vi "Infinite Message Manager - Core.vi"(6 "Infinite Message Selector":T1, 7 "Msg ID":string, 8 "error in (no error)":errorcluster, 9 "Tau parameter":string, 10 "Actor Framework:Message":refnum<class "Message.lvclass">, 11 "Ancestor in":refnum<class "Ancestor.lvclass">) -> (0 "error out":errorcluster, 2 "Exists?":bool, 3 "Ancestor out":refnum<class "Ancestor.lvclass">)   [LabVIEW 2026, in "TALOS.lvlib" / "Ancestor.lvlib" / "Ancestor.lvclass"]
doc: "This VI start the infinite messaging to periodically check the message given in input. It grabs the notifier so to be able to stop it afterwards."
uses:
  Ancestor.lvclass
  builds/Actor Framework PPL/Actor Framework.lvlibp/1abvi3w/vi.lib/ActorFramework/Message/Message.lvclass
  C:/LabVIEW Code/TALOS/builds/Actor Framework PPL/Actor Framework.lvlibp/1abvi3w/vi.lib/ActorFramework/Actor/Actor.lvclass
  Infinite Message Selector.ctl
  Ancestor.lvclass/Ancestor.ctl
  builds/Actor Framework PPL/Actor Framework.lvlibp/1abvi3w/vi.lib/ActorFramework/Time-Delayed Send Message/Time-Delay Override Options.ctl
  FGV/Error Memory/Get Error Description.vi
  Support VIs/Get PC name.vi
  Read ID.vi
  Support VIs/Get Class Name.vi
  Support VIs/Circus Root Path.vi
  FGV/Error Memory/Error Memory Core.vi
  <vilib>/AdvancedString/Delimited String to 1D String Array.vi
  <vilib>/AdvancedString/Delimited String to 1D String Array (string).vi
  FGV/Error Memory/Error Crt Lvl checker.vi
  FGV/Error Memory/Error Memory Core.vi/40c8088d-b597-4017-91af-faa98e00292e.vi
  FGV/Error Memory/Error Memory Core.vi/d4a3ab98-063c-4e44-b43d-fbdcfe6c2be2.vi
  Support VIs/Global Memory.vi
  <vilib>/Utility/LVClass/Get LV Class Name.vi
  Support VIs/Is in Packed Library.vi
  Support VIs/TALOS Root path.vi
  Support VIs/Read CSV worksheet.vi
  Support VIs/Global Constants.vi
  <vilib>/Utility/error.llb/General Error Handler.vi
  <vilib>/Utility/config.llb/Open Config Data.vi
  <vilib>/Utility/config.llb/Get Section Names.vi
  <vilib>/Utility/config.llb/Get Key Names.vi
  <vilib>/Utility/config.llb/Read Key.vi
  <vilib>/Utility/config.llb/Read Key (String).vi
  <vilib>/Utility/config.llb/Close Config Data.vi
  Support VIs/Error Log.vi
  <vilib>/Comparison/Equal/Equal Functor/Equal Functor.lvclass
  builds/Actor Framework PPL/Actor Framework.lvlibp
  builds/Actor Framework PPL/Actor Framework.lvlibp/1abvi3w/vi.lib/ActorFramework/Actor/Actor.lvclass
  TALOS.lvlib
  <userlib>/_OpenG.lib/lvdata/lvdata.llb/openg_variant.lvlib
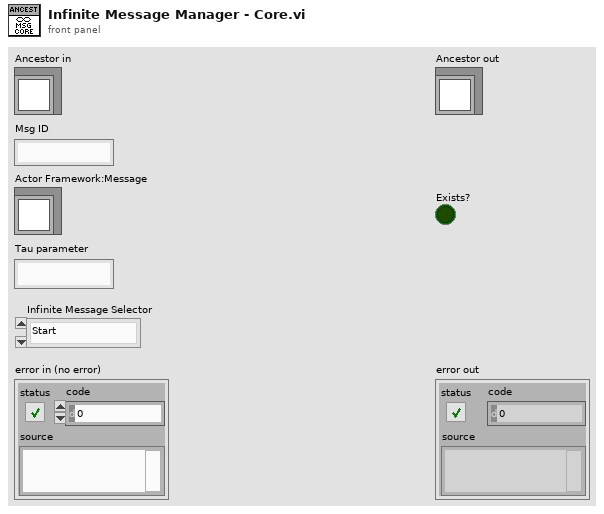
[diagram p1: front panel]
types:
  T1 = typedef "TALOS.lvlib/Ancestor.lvlib/Ancestor.lvclass/Infinite Message Selector.ctl" = enum16{"Start", "Stop", "Check", "Flush (Stop all)", "Init"}
  T2 = typedef "Actor Framework.lvlibp/Time-Delay Override Options.ctl" = enum16{"Send next copy now", "Skip next scheduled copy", "Send next copy now and stop all further copies", "Stop all further copies"}
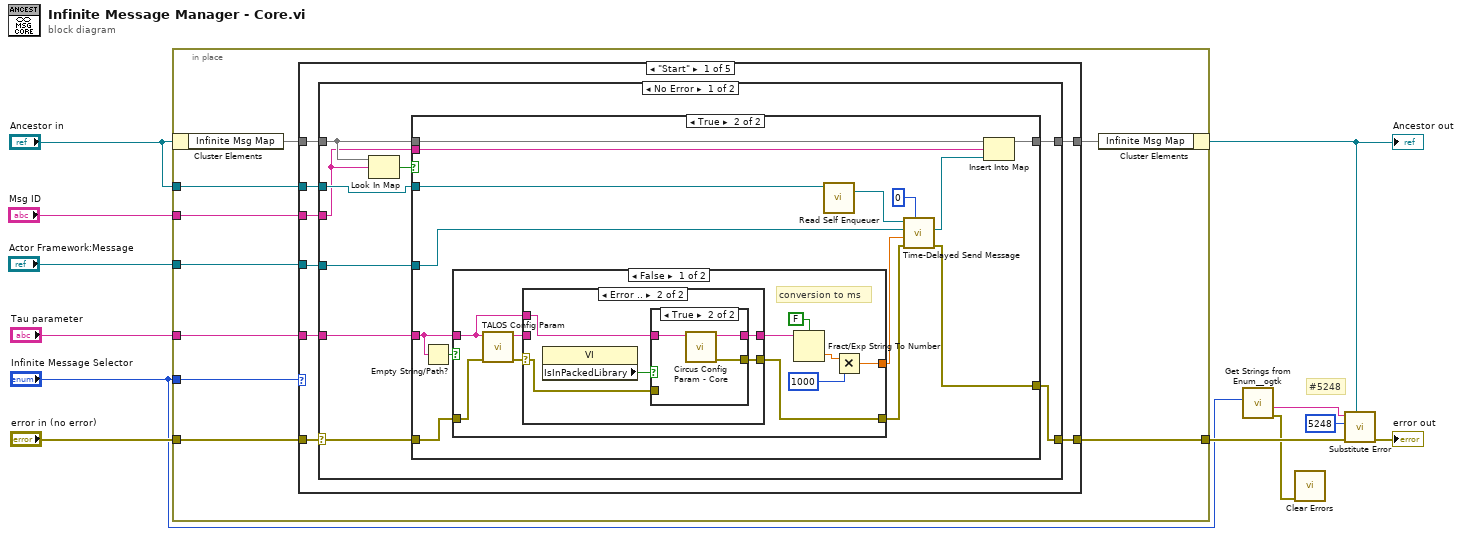
[diagram p0: block diagram]
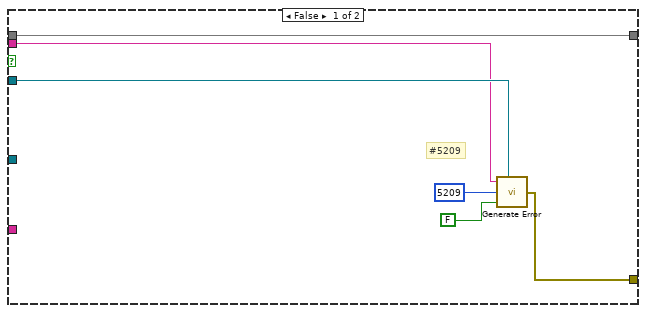
[diagram p2: hidden frame]
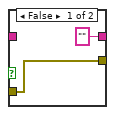
[diagram p4: hidden frame]
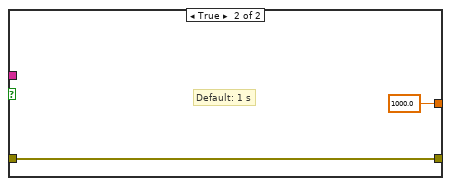
[diagram p5: hidden frame]
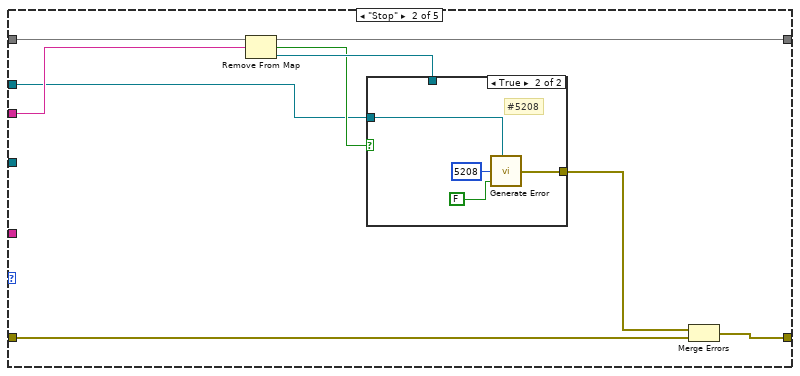
[diagram p7: hidden frame]
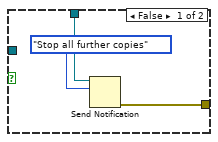
[diagram p8: hidden frame]
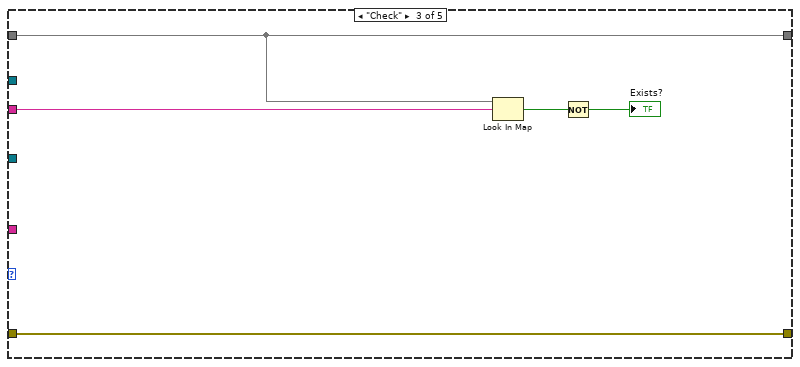
[diagram p9: hidden frame]
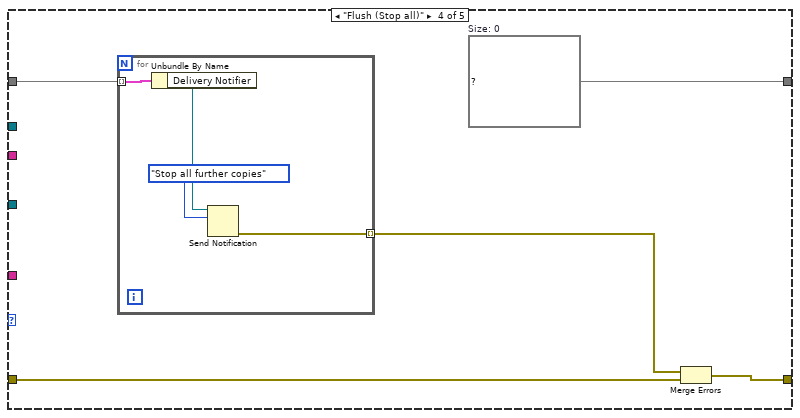
[diagram p10: hidden frame]
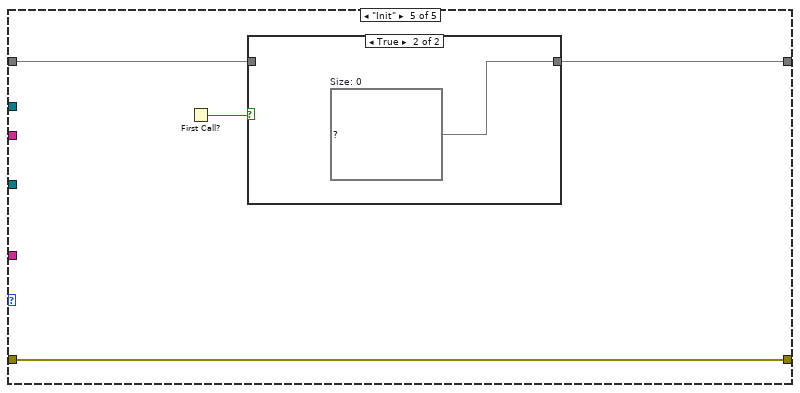
[diagram p11: hidden frame]
diagram:
  # "#5248"
  n1 = in-place {
    in-place-border: "error in (no error)" -> [w13]
    in-place-border: "Actor Framework:Message" -> [w14]
    in-place-border: "Tau parameter" -> [w21]
    in-place-border: "Infinite Message Selector" -> [w20]
    in-place-border: [w19] -> w7
    in-place-border: "Ancestor in" -> [w16]
    in-place-border: "Msg ID" -> [w15]
    n2 = in-place-cluster #1("Ancestor in") -> ("Infinite Msg Map"=w18:map{string, refnum<notifier>})
    n3 = case shown="\"Start\"" w20 {
      tunnel: w16 -> [w29 w87 _ _ _]
      tunnel: [w28 w86 w101 w107 w117] -> w19
      tunnel: [w25 w92 w105 w109 w118] -> w17
      tunnel: w18 -> [w23 w91 w105 w110 w115]
      tunnel: w14 -> [w26 _ _ _ _]
      tunnel: w21 -> [w27 _ _ _ _]
      tunnel: w15 -> [w22 w88 w104 _ _]
      tunnel: w13 -> [w24 w85 w101 w106 w117]
      frame "Start" {
        n4 = case shown="No Error" w24 {
          selector: w24 -> [w33 w84]
          tunnel: w29 -> [w38 _]
          tunnel: [w37 w84] -> w28
          tunnel: w27 -> [w36 _]
          tunnel: w26 -> [w35 _]
          tunnel: [w34 w83] -> w25
          tunnel: w23 -> [w32 w83]
          tunnel: w22 -> [w31 _]
          frame No Error {
            n5 = Look In Map(map=w32, key=w31) -> (key not found?=w30:bool)  [unwired: 1 in, 1 out]
            n6 = case shown="True" w30 {
              tunnel: w38 -> [w40 w55]
              tunnel: [w41 w54] -> w37
              tunnel: w36 -> [_ w45]
              tunnel: w35 -> [_ w53]
              tunnel: [w44 w51] -> w34
              tunnel: w33 -> [_ w50]
              tunnel: w32 -> [w44 w49]
              tunnel: w31 -> [w39 w48]
              frame False {
                # "#5209"
                n7 = call "Generate Error.vi"("Optional String"=w39, "Class"=w40, "Error Code"=5209, "Error/Warning"=FALSE) -> ("error out"=w41:errorcluster)  [unwired: 3 in]
              }
              frame True {
                n8 = Empty String/Path?(string/path=w45) -> (empty?=w46:bool)
                n9 = case shown="False" w46 {
                  tunnel: [w68 1000.0] -> w57
                  tunnel: w50 -> [w66 w82]
                  tunnel: [w63 w82] -> w47
                  tunnel: w45 -> [w62 _]
                  frame False {
                    # "conversion to ms"
                    n10 = call "TALOS Config Param.vi"("error in (no error)"=w66, "Parameter Name"=w62) -> ("error out"=w65:errorcluster, "Output"=w64:string)  [unwired: 8 in]
                    n11 = case shown="Error .." w65 {
                      selector: w65 -> [w70 w73]
                      tunnel: w64 -> [w69 _]
                      tunnel: [w70 w72] -> w63
                      tunnel: [w69 w74] -> w61
                      tunnel: w62 -> [_ w71]
                      frame No Error {
                      }
                      frame Error {
                        n12 = property class="VI"() -> ("IsInPackedLibrary"=w75:bool)  [unwired: 2 in, 2 out]
                        n13 = case shown="True" w75 {
                          tunnel: ["" ("Output") w79] -> w74
                          tunnel: w73 -> [w77 _]
                          tunnel: [w77 w80] -> w72
                          tunnel: w71 -> [_ w78]
                          frame False {
                          }
                          frame True {
                            n14 = call "Circus Config Param - Core.vi"("Parameter Name"=w78) -> ("error out"=w80:errorcluster, "Output"=w79:string)  [unwired: 9 in]
                          }
                        }
                      }
                    }
                    n15 = Fract/Exp String To Number(use system decimal point (T)=FALSE, string=w61) -> (number=w60:dbl)  [unwired: 2 in, 1 out]
                    n16 = Multiply(x=w60, y=1000) -> (x*y=w68:dbl)
                  }
                  frame True {
                    # "Default: 1 s"
                  }
                }
                n17 = call "Read Self Enqueuer.vi"("Actor"=w55) -> ("Self Enqueuer"=w56:refnum<class "Message Enqueuer.lvclass">)  [unwired: 10 in]
                n18 = call "Time-Delayed Send Message.vi"("# Copies (0 = infinite repeat)"=u32 0, "error in (no error)"=w47, "Milliseconds To Wait"=w57, "Message"=w53, "Message Enqueuer"=w56) -> ("error out"=w54:errorcluster, "Delivery Notifier"=w52:refnum<notifier>)  [unwired: 5 in]
                n19 = Insert Into Map(map in=w49, key=w48, value=w52) -> (map out=w51:map{string, refnum<notifier>})  [unwired: 2 out]
              }
            }
          }
          frame Error {
          }
        }
      }
      frame "Stop" {
        n20 = Remove From Map(10:w88, 11:w91) -> (1:w90:refnum<notifier>, 2:w89:bool, 3:w92:map{string, refnum<notifier>})
        n21 = case shown="True" w89 {
          tunnel: [w95 w100] -> w93
          tunnel: w90 -> [w94 _]
          tunnel: w87 -> [_ w97]
          frame False {
            n22 = Send Notification(notification=Time-Delay_Override_Options."Stop all further copies", notifier=w94) -> (error out=w95:errorcluster)  [unwired: 1 in, 1 out]
          }
          frame True {
            # "#5208"
            n23 = call "Generate Error.vi"("Class"=w97, "Error Code"=5208, "Error/Warning"=FALSE) -> ("error out"=w100:errorcluster)  [unwired: 4 in]
          }
        }
        n24 = Merge Errors(w93, w85) -> (w86:errorcluster)
      }
      frame "Check" {
        n25 = Look In Map(map=w105, key=w104) -> (key not found?=w103:bool)  [unwired: 1 in, 1 out]
        n26 = Not(x=w103) -> (.not. x?=→"Exists?":bool)
      }
      frame "Flush (Stop all)" {
        w109 = map{string, refnum<notifier>} {}  # Size: 0
        n27 = for {
          tunnel: w110 -> [w113] mode=indexing
          tunnel: [w111] -> w108 mode=indexing
          n28 = Unbundle By Name(w113) -> ("Delivery Notifier"=w112:refnum<notifier>)
          n29 = Send Notification(notification=Time-Delay_Override_Options."Stop all further copies", notifier=w112) -> (error out=w111:errorcluster)  [unwired: 1 in, 1 out]
        }
        n30 = Merge Errors(w108, w106) -> (w107:errorcluster)
      }
      frame "Init" {
        n31 = First Call?() -> (First Call?: T/F=w116:bool)
        n32 = case shown="True" w116 {
          tunnel: [w119 w120] -> w118
          tunnel: w115 -> [w119 _]
          frame False {
            # "To be sure to clean it only once, at startup."
          }
          frame True {
            w120 = map{string, refnum<notifier>} {}  # Size: 0
          }
        }
      }
    }
    n33 = in-place-cluster #1("Infinite Msg Map"=w17) -> (w5:refnum<class "Ancestor.lvclass">)
  }
  "Ancestor out" <- w5
  n34 = call <userlib>:"Get Strings from Enum__ogtk.vi"("Enum"="Infinite Message Selector") -> ("error out"=w2:errorcluster, "String Value"=w1:string)  [unwired: 7 in, 2 out]
  n35 = call <vilib>:"Clear Errors.vi"("error in (no error)"=w2) -> ()  [unwired: 5 in, 2 out]
  n36 = call "Substitute Error.vi"("LabVIEW Object"=w5, "error in (no error)"=w7, "Error Code"=5248, "Optional String"=w1) -> ("error out"=→"error out":errorcluster)  [unwired: 7 in]
